vi "UnoLoopbackTesterv6.vi"() -> ()   [LabVIEW 2009]
uses:
  <vilib>/Instr/_visa.llb/VISA Configure Serial Port (Instr).vi
panel:
  in  "stop":bool
  in  "System":enum32{"Main", "Serial Terminal"}(tab)=enum."Serial Terminal"
  out "Outgoing Messages":string
  in  "Send":bool
  in  "Input":string
  out "Incoming Messages":string
  in  "VISA resource name":refnum<visa-resource-name>
  in  "baud rate (9600)":u32=9600
  in  "data bits (8)":u16=8 min=5 max=8 step=1
  in  "parity (0:none)":enum16{"None", "Odd", "Even", "Mark", "Space"}(ring)
  in  "stop bits (10: 1 bit)":u16(ring)=10 items=["1.0"=10, "1.5"=15, "2.0"=20]
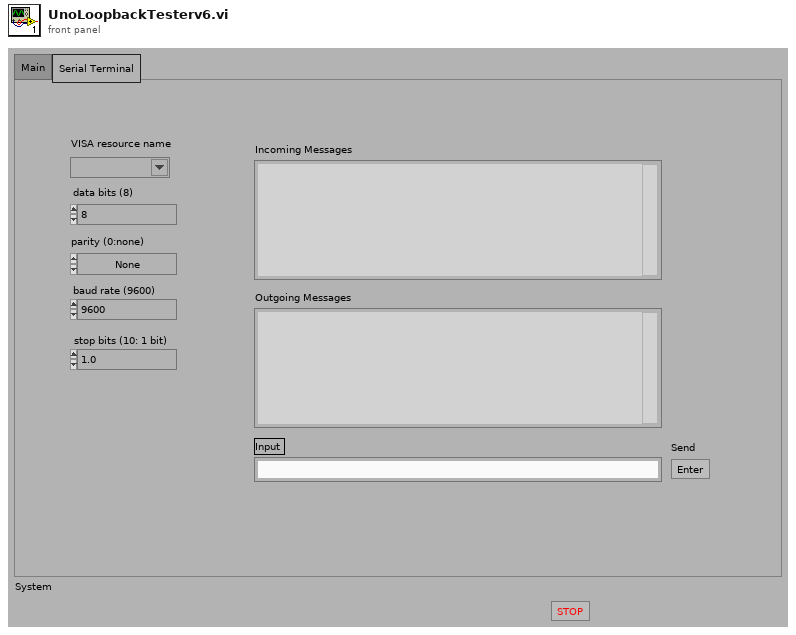
[diagram p1: front panel]
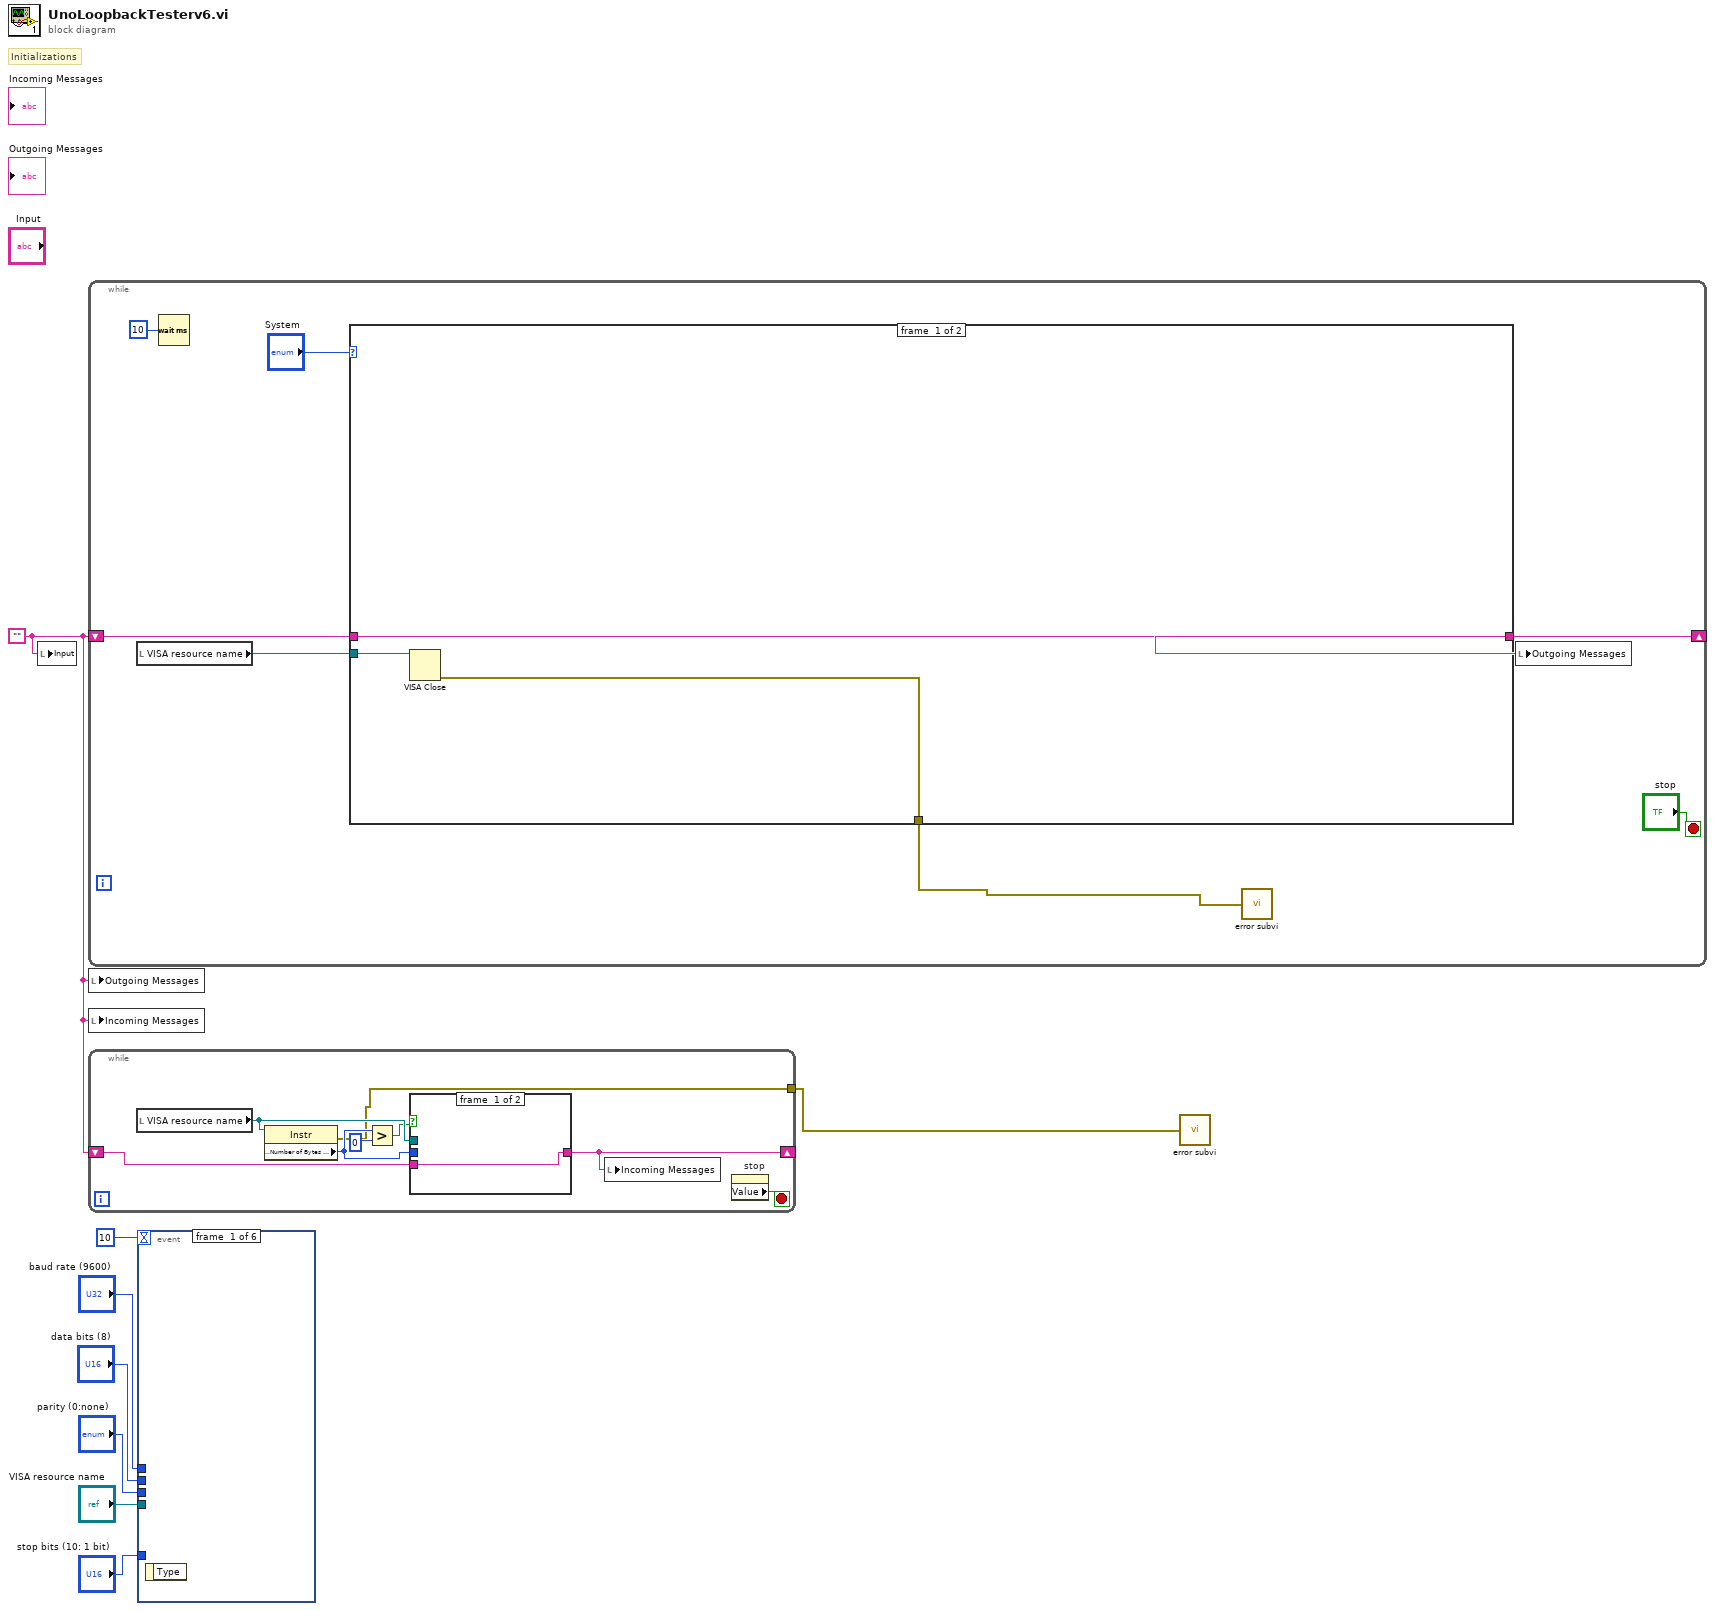
[diagram p0: block diagram]
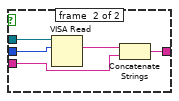
[diagram p2: hidden frame]
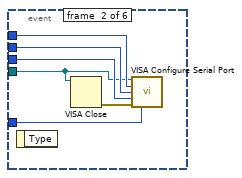
[diagram p3: hidden frame]
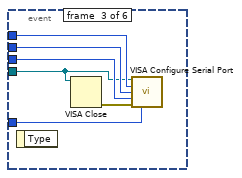
[diagram p4: hidden frame]
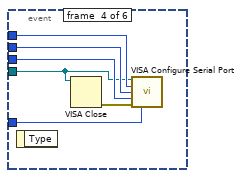
[diagram p5: hidden frame]
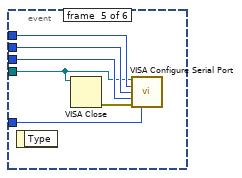
[diagram p6: hidden frame]
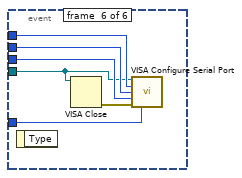
[diagram p7: hidden frame]
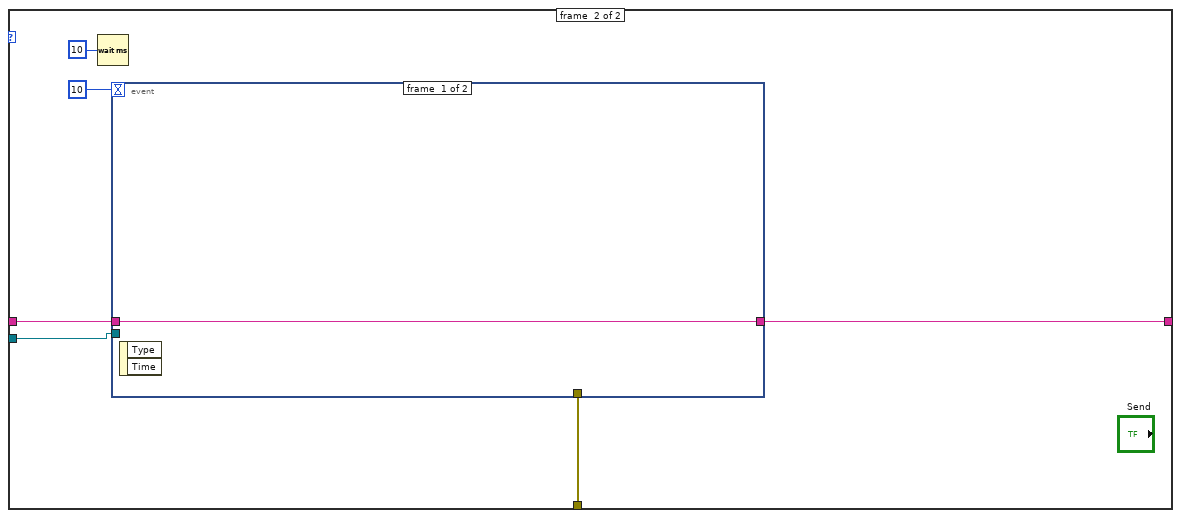
[diagram p8: hidden frame]
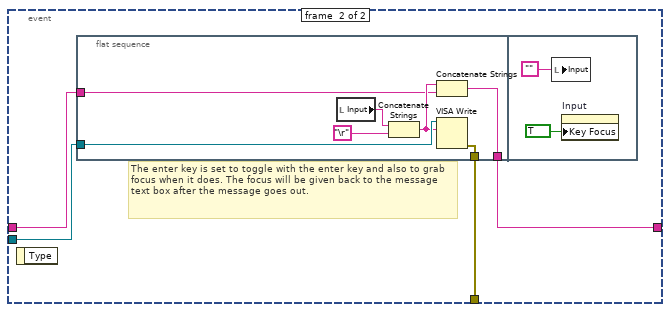
[diagram p9: hidden frame]
diagram:
  w2 = ""
  # "Initializations"
  n1 = local write "Input"(w2) -> ()
  n2 = while {
    shift-right: [w11] -> _
    shift-left: w2 -> [w12]
    stop <- "stop" stop-if-true
    n3 = local read "VISA resource name"() -> (w13:refnum<visa-resource-name>)
    n4 = Wait (ms)(milliseconds to wait=u32 10) -> ()  [unwired: 1 out]
    n5 = case shown="\"Serial Terminal\"" "System" {
      tunnel: w13 -> [w18 w22]
      tunnel: [w17 w21] -> w11
      tunnel: w12 -> [w17 w20]
      tunnel: [w16 w19] -> w9
      frame #0 {
        n6 = VISA Close(VISA resource name=w18) -> (error out=w16:errorcluster)  [unwired: 1 in]
      }
      frame #1 {
        n7 = Wait (ms)(milliseconds to wait=u32 10) -> ()  [unwired: 1 out]
        n8 = event shown="[1] \"Send\": Value Change" {
          selector: _ -> [_ _]
          dyn-events: _ -> [_ _]
          timeout: 10 -> [_ _]
          tunnel: w22 -> [_ w29]
          tunnel: [w25 w27] -> w21
          tunnel: w20 -> [w25 w28]
          tunnel: [_ w26] -> w19
          event #0 {
            n9 = event-data() -> ()  [unwired: 1 in, 2 out]
          }
          event #1 {
            # "The enter key is set to toggle with the enter key and also to grab focus when it does. The focus will be given back to the message text box after the message goes out."
            n10 = event-data() -> ()  [unwired: 1 in, 1 out]
            n11 = flat-sequence {
              tunnel: w29 -> [w34]
              tunnel: w28 -> [w32]
              tunnel: [w31] -> w27
              tunnel: [w30] -> w26
              frame #0 {
                n12 = local read "Input"() -> (w36:string)
                n13 = Concatenate Strings(w36, "\r") -> (w33:string)
                n14 = Concatenate Strings(w33, w32) -> (w31:string)
                n15 = VISA Write(VISA resource name=w34, write buffer=w33) -> (error out=w30:errorcluster)  [unwired: 1 in, 2 out]
              }
              frame #1 {
                n16 = local write "Input"("") -> ()
                n17 = property on="Input" class="Str"("Key Focus"=TRUE) -> ()  [unwired: 2 in, 2 out]
              }
            }
          }
        }
      }
    }
    n18 = call "error subvi.vi"("error out"=w9) -> ()
    n19 = local write "Outgoing Messages"(w11) -> ()
  }
  n20 = local write "Outgoing Messages"(w2) -> ()
  n21 = local write "Incoming Messages"(w2) -> ()
  n22 = while {
    shift-right: [w40] -> _
    shift-left: w2 -> [w41]
    tunnel: [w39] -> w1
    stop <- w45 stop-if-true
    n23 = local read "VISA resource name"() -> (w46:refnum<visa-resource-name>)
    n24 = property class="Instr"(reference=w46) -> (error out=w39:errorcluster, "Serial Settings:Number of Bytes at Serial Port"=w42:u32)  [unwired: 1 in, 1 out]
    n25 = Greater?(x=w42, y=u32 0) -> (0:w43:bool)
    n26 = case shown="False" w43 {
      tunnel: w46 -> [_ w52]
      tunnel: w42 -> [_ w51]
      tunnel: w41 -> [w47 w48]
      tunnel: [w47 w49] -> w40
      frame #0 {
      }
      frame #1 {
        n27 = VISA Read(VISA resource name=w52, byte count=w51) -> (read buffer=w50:string)  [unwired: 1 in, 3 out]
        n28 = Concatenate Strings(w50, w48) -> (w49:string)
      }
    }
    n29 = local write "Incoming Messages"(w40) -> ()
    n30 = property on="stop" class="Bool (strict)"() -> ("Value"=w45:bool)  [unwired: 2 in, 2 out]
  }
  n31 = event shown="[5] \"stop bits (10: 1 bit)\": Value Change" {
    selector: _ -> [_ _ _ _ _ _]
    dyn-events: _ -> [_ _ _ _ _ _]
    timeout: 10 -> [_ _ _ _ _ _]
    tunnel: "VISA resource name" -> [_ w53 w59 w65 w71 w77]
    tunnel: "baud rate (9600)" -> [_ w58 w64 w70 w76 w82]
    tunnel: "data bits (8)" -> [_ w57 w63 w69 w75 w81]
    tunnel: "parity (0:none)" -> [_ w56 w62 w68 w74 w80]
    tunnel: "stop bits (10: 1 bit)" -> [_ w55 w61 w67 w73 w79]
    event #0 {
      n32 = event-data() -> ()  [unwired: 1 in, 1 out]
    }
    event #1 {
      n33 = event-data() -> ()  [unwired: 1 in, 1 out]
      n34 = VISA Close(VISA resource name=w53) -> (error out=w54:errorcluster)  [unwired: 1 in]
      n35 = call-poly "VISA Configure Serial Port"("VISA resource name"=w53, "baud rate (9600)"=w58, "data bits (8)"=w57, "parity (0:none)"=w56, "error in (no error)"=w54, "stop bits (10: 1 bit)"=w55) -> ()  [unwired: 8 in, 2 out]
    }
    event #2 {
      n36 = event-data() -> ()  [unwired: 1 in, 1 out]
      n37 = VISA Close(VISA resource name=w59) -> (error out=w60:errorcluster)  [unwired: 1 in]
      n38 = call-poly "VISA Configure Serial Port"("VISA resource name"=w59, "baud rate (9600)"=w64, "data bits (8)"=w63, "parity (0:none)"=w62, "error in (no error)"=w60, "stop bits (10: 1 bit)"=w61) -> ()  [unwired: 8 in, 2 out]
    }
    event #3 {
      n39 = event-data() -> ()  [unwired: 1 in, 1 out]
      n40 = VISA Close(VISA resource name=w65) -> (error out=w66:errorcluster)  [unwired: 1 in]
      n41 = call-poly "VISA Configure Serial Port"("VISA resource name"=w65, "baud rate (9600)"=w70, "data bits (8)"=w69, "parity (0:none)"=w68, "error in (no error)"=w66, "stop bits (10: 1 bit)"=w67) -> ()  [unwired: 8 in, 2 out]
    }
    event #4 {
      n42 = event-data() -> ()  [unwired: 1 in, 1 out]
      n43 = VISA Close(VISA resource name=w71) -> (error out=w72:errorcluster)  [unwired: 1 in]
      n44 = call-poly "VISA Configure Serial Port"("VISA resource name"=w71, "baud rate (9600)"=w76, "data bits (8)"=w75, "parity (0:none)"=w74, "error in (no error)"=w72, "stop bits (10: 1 bit)"=w73) -> ()  [unwired: 8 in, 2 out]
    }
    event #5 {
      n45 = event-data() -> ()  [unwired: 1 in, 1 out]
      n46 = VISA Close(VISA resource name=w77) -> (error out=w78:errorcluster)  [unwired: 1 in]
      n47 = call-poly "VISA Configure Serial Port"("VISA resource name"=w77, "baud rate (9600)"=w82, "data bits (8)"=w81, "parity (0:none)"=w80, "error in (no error)"=w78, "stop bits (10: 1 bit)"=w79) -> ()  [unwired: 8 in, 2 out]
    }
  }
  n48 = call "error subvi.vi"("error out"=w1) -> ()
